vi "End Array by Value.vi"(8 "Error In":errorcluster, 11 "Reader In":refnum<class "Reader.lvclass">) -> (0 "Error Out":errorcluster, 3 "Reader Out":refnum<class "Reader.lvclass">)   [LabVIEW 2019, in "LabPack.lvlib" / "Reader.lvclass"]
uses:
  Reader.lvclass
  Reader.lvclass/Reader.ctl
  Public/Status/Read Status.vi
  Public/Status/Read Status Message.vi
  Public/Status/Read Is Error.vi
  Utility/Status Code.vi
  <vilib>/Utility/error.llb/Error Cluster From Error Code.vi
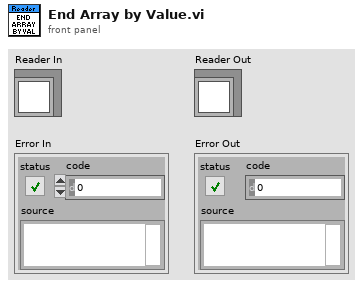
[diagram p1: front panel]
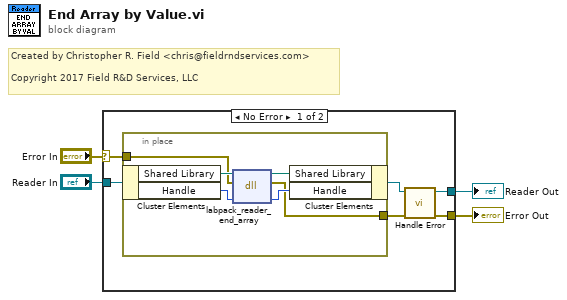
[diagram p0: block diagram]
diagram:
  # "Created by Christopher R. Field <chris@fieldrndservices.com>\n\nCopyright 2017 Field R&D Services, LLC"
  n1 = case shown="No Error" "Error In" {
    selector: "Error In" -> [w9 w18]
    tunnel: "Reader In" -> [w10 w17]
    tunnel: [w5 w18] -> w2
    tunnel: [w7 w17] -> w1
    frame No Error {
      n2 = in-place {
        in-place-border: w9 -> [w12]
        in-place-border: [w11] -> w6
        n3 = in-place-cluster #1(w10) -> ("Shared Library"=w16:path, "Handle"=w14:u64)
        n4 = dll-call lib="D:/Users/cfield/Code/MessagePack/LabPack/LabVIEW/trunk/src/LabPack/Private/labpack-x64.dll" fn="labpack_reader_end_array"(path in=w16, error in=w12, "reader"=w14) -> (path out=w15:path, error out=w11:errorcluster, "reader"=w13:u64)  [unwired: 2 in]
        n5 = in-place-cluster #1("Shared Library"=w15, "Handle"=w13) -> (w8:refnum<class "Reader.lvclass">)
      }
      n6 = call "Handle Error.vi"("Error In"=w6, "Reader In"=w8) -> ("Error Out"=w5:errorcluster, "Reader Out"=w7:refnum<class "Reader.lvclass">)  [unwired: 8 in]
    }
    frame Error {
    }
  }
  "Error Out" <- w2
  "Reader Out" <- w1
